vi "Test Bernoulli Trial.vi"() -> ()   [LabVIEW 2015]
panel:
  out "sum":i16
  in  "Nrand":i32=1
  out "error out":errorcluster
  out "y value":dbl[](array[numeric])=[0.0, 0.5877853083428206, 0.9510565591138008, 0.9510564520671484, 0.5877850280910549, -3.464102066193935e-07, -0.5877855885945158, -0.9510566661603391, -0.9510563450203818, -0.5877847478392194, 6.928204132387453e-07] format="%0.2f"
  in  "expression":string="bernrnd(1,[0 1 2],[0 0.5 1])"
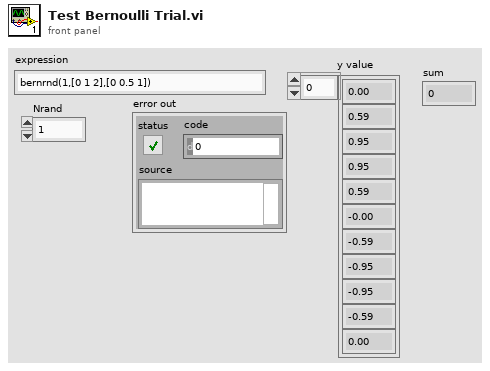
[diagram p1: front panel]
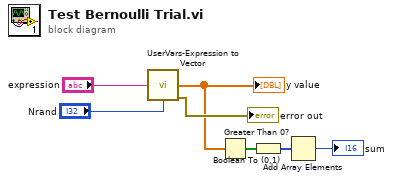
[diagram p0: block diagram]
diagram:
  n1 = call "UserVars-Expression to Vector.vi"("Expr"="expression", "Nrand"="Nrand") -> ("Values"=w4:dbl[], "error out"=→"error out":errorcluster)  [unwired: 12 in]
  "y value" <- w4
  n2 = Greater Than 0?(x=w4) -> (x > 0?=w3:bool[])
  n3 = Boolean To (0,1)(Boolean=w3) -> (0, 1=w2:i16[])
  n4 = Add Array Elements(numeric array=w2) -> (sum=→"sum":i16)
